vi "_Write.vi"(8 "error in (no error)":errorcluster, 10 "Data":string, 11 "FileStream in":refnum<class "FileStream.lvclass">) -> (0 "error out":errorcluster, 3 "FileStream out":refnum<class "FileStream.lvclass">)   [LabVIEW 2020, in "Stream.lvlib" / "FileStream.lvclass"]
uses:
  FileStream.lvclass
  FileStream.lvclass/FileStream.ctl
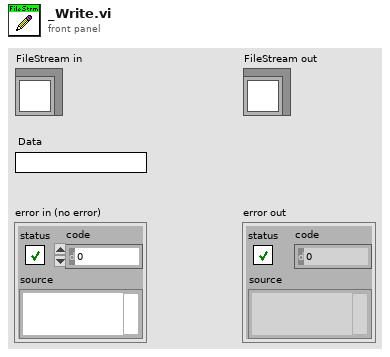
[diagram p1: front panel]
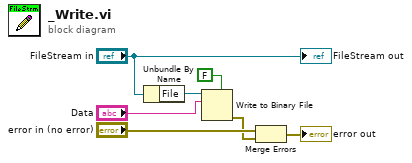
[diagram p0: block diagram]
diagram:
  n1 = Unbundle By Name("FileStream in") -> ("File"=w5:refnum<file>)
  n2 = Write to Binary File(file (use dialog)=w5, data="Data", 5:FALSE ("prepend array or string size? (T)")) -> (error out=w3:errorcluster)  [unwired: 3 in, 2 out]
  n3 = Merge Errors("error in (no error)", w3) -> (→"error out":errorcluster)
  "FileStream out" <- "FileStream in"
